vi "repainter.vi"(1 "Array":cluster{"X":i32, "Y":i32}[][](array[cluster]), 2 "Selected Line":i32=-1) -> (0 "Picture":picture)   [LabVIEW 2017]
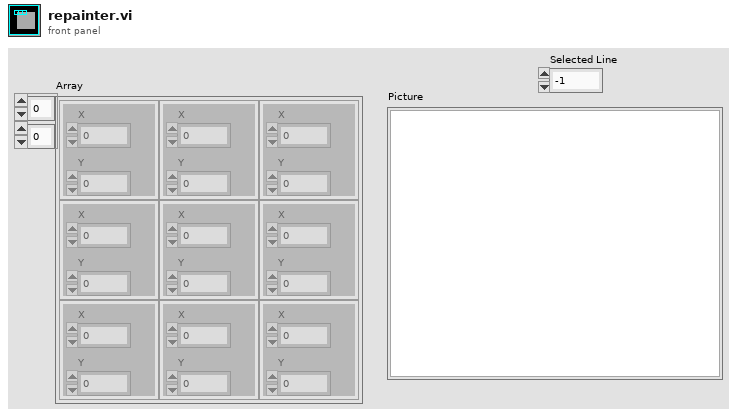
[diagram p1: front panel]
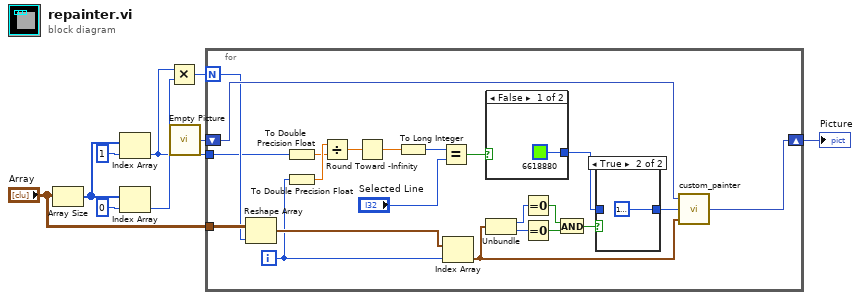
[diagram p0: block diagram]
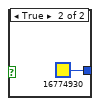
[diagram p3: hidden frame]
diagram:
  n1 = Array Size(array="Array") -> (size(s)=w5:i32[])
  n2 = Index Array(array=w5, index=1) -> (element=w2:i32)
  n3 = Index Array(array=w5, index=0) -> (element=w3:i32)
  n4 = Multiply(x=w2, y=w3) -> (x*y=w4:i32)
  n5 = call "Empty Picture"() -> ("empty picture"=w9:picture)
  n6 = for {
    N: w4 -> [w27]
    shift-right: [w30] -> w8
    shift-left: w9 -> [w31]
    tunnel: "Array" -> [w29]
    tunnel: w2 -> [w20]
    i -> [w26]
    n7 = Reshape Array(w29, w27) -> (w28:cluster{"X":i32, "Y":i32}[])
    n8 = To Double Precision Float(number=w20) -> (double precision float=w24:dbl)
    n9 = To Double Precision Float(number=w26) -> (double precision float=w25:dbl)
    n10 = Divide(x=w25, y=w24) -> (x/y=w19:dbl)
    n11 = Round Toward -Infinity(1:w19) -> (0:w18:dbl)
    n12 = To Long Integer(number=w18) -> (32bit integer=w22:i32)
    n13 = Equal?(x=w22, y="Selected Line") -> (x = y?=w21:bool)
    n14 = Index Array(array=w28, index=w26) -> (element=w15:cluster{"X":i32, "Y":i32})
    n15 = case shown="False" w21 {
      tunnel: [u32 6618880 ("color(black)") u32 16774930 ("color(black)")] -> w16
      frame False {
      }
      frame True {
      }
    }
    n16 = Unbundle(w15) -> ("X"=w14:i32, "Y"=w13:i32)
    n17 = Equal To 0?(x=w14) -> (x = 0?=w11:bool)
    n18 = Equal To 0?(x=w13) -> (x = 0?=w12:bool)
    n19 = And(x=w11, y=w12) -> (x .and. y?=w10:bool)
    n20 = case shown="True" w10 {
      tunnel: [w32 u32 16777228 ("color(black)")] -> w17
      tunnel: w16 -> [w32 _]
      frame False {
      }
      frame True {
      }
    }
    n21 = call "custom_painter.vi"("Point"=w15, "Color"=w17, "Picture in"=w31) -> ("Picture out"=w30:picture)
  }
  "Picture" <- w8
